vi "Pkt - Get SysDef Version.vi"(8 "error in (no error)":errorcluster, 11 "Packet Ref In":T1=18446744073709551615 format="%.0x") -> (0 "error out":errorcluster, 1 "Version String":string, 2 "Encoded Version":u64 format="%016x", 3 "Packet Ref out":T1=18446744073709551615 format="%.0x")   [LabVIEW 2016, in "UDP-Custom-Device System Explorer.lvlib"]
uses:
  UDP-Custom-Device System Explorer.lvlib
  <vilib>/NI Veristand/Custom Device API/Custom Device Item Ref.ctl
  NationalInstruments.VeriStand.SystemDefinitionAPI
  <vilib>/NI Veristand/Custom Device Offline API/Custom Device Offline API.lvlib
  <vilib>/NI VeriStand/Custom Device API/Custom Device API.lvlib
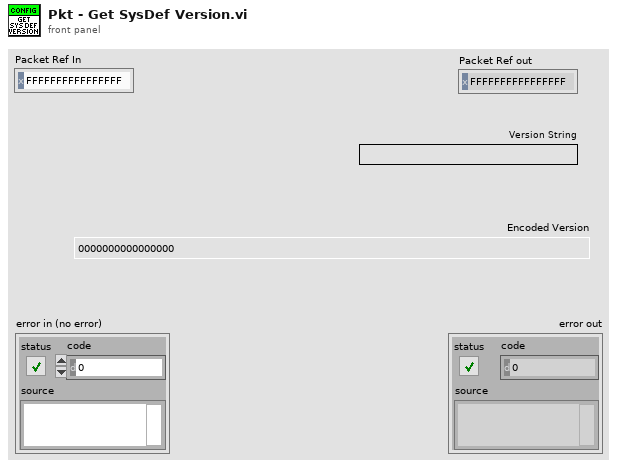
[diagram p1: front panel]
types:
  T1 = typedef "Custom Device API.lvlib/Custom Device Item Ref.ctl" = u64
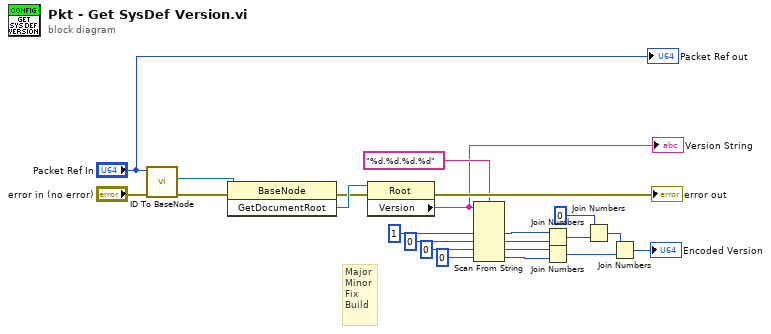
[diagram p0: block diagram]
diagram:
  # "Major\nMinor\nFix\nBuild"
  n1 = call <vilib>:"ID To BaseNode.vi"("error in (no error)"="error in (no error)", "ID in"="Packet Ref In") -> ("error out"=w19:errorcluster, "BaseNode"=w20:refnum<k24>)  [unwired: 7 in, 1 out]
  n2 = invoke class="BaseNode" method="GetDocumentRoot"(reference=w20, error in=w19) -> (error out=w17:errorcluster, "GetDocumentRoot"=w18:refnum<k24>)  [unwired: 1 in, 1 out]
  n3 = property class="Root"(reference=w18, error in=w17) -> (error out=→"error out":errorcluster, "Version"=w1:string)  [unwired: 1 out]
  "Version String" <- w1
  n4 = Scan From String(format string="%d.%d.%d.%d", input string=w1, default 1=u8 1 ("default value 1"), default 2=u8 0 ("default value 2"), default 3=u16 0 ("default value 3"), default 4=u16 0 ("default value 4")) -> (output 1=w10:u8, output 2=w9:u8, output 3=w6:u16, output 4=w5:u16)  [unwired: 2 in, 3 out]
  n5 = Join Numbers(hi=w10, lo=w9) -> ((hi.lo)=w7:u16)
  n6 = Join Numbers(hi=w6, lo=w5) -> ((hi.lo)=w3:u32)
  n7 = Join Numbers(hi=u16 0 ("default value 2"), lo=w7) -> ((hi.lo)=w4:u32)
  n8 = Join Numbers(hi=w4, lo=w3) -> ((hi.lo)=→"Encoded Version":u64)
  "Packet Ref out" <- "Packet Ref In"
